vi "maxmin.vi"(3 "Numeric 2":dbl, 5 "Numeric":dbl) -> (0 "Smallest":dbl, 2 "greatest":dbl)   [LabVIEW 2014]
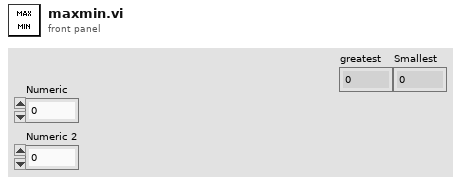
[diagram p1: front panel]
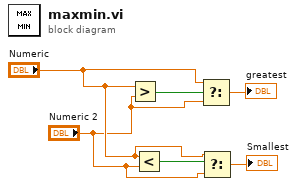
[diagram p0: block diagram]
diagram:
  n1 = Greater?(x="Numeric", y="Numeric 2") -> (0:w6:bool)
  n2 = Less?(x="Numeric", y="Numeric 2") -> (x < y?=w4:bool)
  n3 = Select(t="Numeric", s=w6, f="Numeric 2") -> (s? t:f=→"greatest":dbl)
  n4 = Select(t="Numeric", s=w4, f="Numeric 2") -> (s? t:f=→"Smallest":dbl)
